vi "Configure PCM Settings.vi"(8 "error in":errorcluster, 11 "Measurement Configuration":T1={"Analog Source Resource Name"="", "IMD Standard"=0, "Custom Low Frequency"=14000.0, "Custom High frequency"=15000.0, "Custom Amplitude Ratio"=1.0, "Amplitude"=-1.0, "Protocol Source Resource Name"="7821\\PCMi 0", "Input range"=2.825, "Number of Words"=19200, "Clock Rate"=12288000, "Latch Delay"=0.0} {"Custom Amplitude Ratio" format="%.1f"; "Custom High frequency" format="%_2p"; "Custom Low Frequency" format="%#_2p"; "Clock Rate" format="%.4p"}) -> (0 "error out":errorcluster, 3 "PCM Input Task out":T2)   [LabVIEW 2021, in "audio_intermodulationDistortionMeasurement.lvlib"]
uses:
  audio_intermodulationDistortionMeasurement.lvlib
  <vilib>/PDM Acquisition Toolkit/host/Classes/Tasks/PCM Input/Controls/DVR PCM Input Task.ctl
  <vilib>/PDM Acquisition Toolkit/host/Classes/Tasks/PCM Input/PCM Input Task.lvclass
  <vilib>/PDM Acquisition Toolkit/host/Classes/Tasks/PDM Tasks/Controls/Acquisition Mode.ctl
  <vilib>/PDM Acquisition Toolkit/shared/controls/PCM Frame Sync Control.ctl
  <vilib>/PDM Acquisition Toolkit/shared/controls/Digital Edge.ctl
  <vilib>/PDM Acquisition Toolkit/shared/controls/PCM Data Format Configuration.ctl
  <vilib>/PDM Acquisition Toolkit/shared/controls/PCM Bit Endianness.ctl
  <vilib>/PDM Acquisition Toolkit/shared/controls/PCM Data Justification.ctl
  <vilib>/PDM Acquisition Toolkit/host/Classes/Session/Controls/Logic Levels.ctl
  <vilib>/PDM Acquisition Toolkit/host/API/Public/Create Tasks/Create PCM Input Task.vi
  <vilib>/PDM Acquisition Toolkit/host/API/Public/Configure/Timing/Configure Timing - PCM Input Slave.vi
  <vilib>/PDM Acquisition Toolkit/host/API/Public/Configure/PDM Channel/Configure Microphone Sensitivity FSPA - PCM Input Task.vi
  <vilib>/PDM Acquisition Toolkit/host/API/PDM Acquisition Toolkit.lvlib
  <vilib>/PDM Acquisition Toolkit/host/Classes/Tasks/PDM Tasks/PDM Task.lvclass
  <vilib>/PDM Acquisition Toolkit/shared/PDM Shared.lvlib
  <vilib>/PDM Acquisition Toolkit/host/Classes/Session/DecoderSession.lvclass
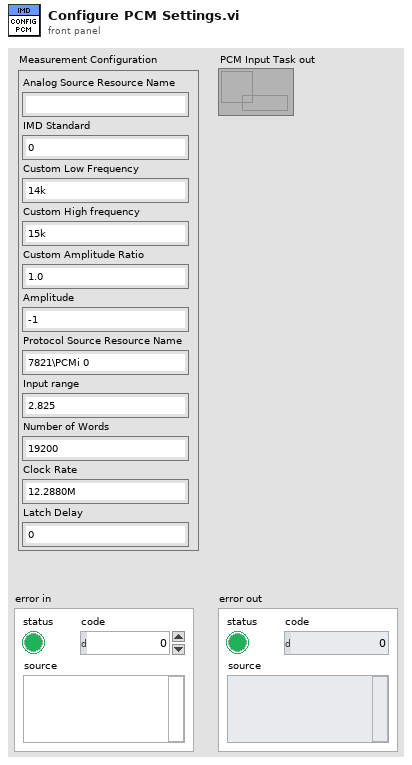
[diagram p1: front panel]
types:
  T1 = cluster{"Analog Source Resource Name":string, "IMD Standard":u16, "Custom Low Frequency":dbl, "Custom High frequency":dbl, "Custom Amplitude Ratio":dbl, "Amplitude":dbl, "Protocol Source Resource Name":string, "Input range":dbl, "Number of Words":i32, "Clock Rate":u32, "Latch Delay":dbl}
  T2 = typedef "PDM Acquisition Class Library.lvlib/PCM Input Task.lvclass/DVR PCM Input Task.ctl" = refnum<data-value>
  T3 = typedef "PDM Acquisition Class Library.lvlib/DecoderSession.lvclass/Logic Levels.ctl" = enum16{"3.3 V", "1.8 V", "1.2 V"}
  T4 = typedef "PDM Shared.lvlib/PCM Data Format Configuration.ctl" = cluster{"Frame Sync Edge for Channel 0":T5, "Channel Count Per Frame":u8, "Channel Length":u16, "Bit Depth":u8, "Channel 0 Offset":u16, "Endianness":T6, "Data Justification":T7}
  T5 = typedef "PDM Shared.lvlib/Digital Edge.ctl" = enum8{"Rising", "Falling"}
  T6 = typedef "PDM Shared.lvlib/PCM Bit Endianness.ctl" = enum16{"MSB First", "LSB First"}
  T7 = typedef "PDM Shared.lvlib/PCM Data Justification.ctl" = enum16{"Left Justified", "Right Justified"}
  T8 = typedef "PDM Shared.lvlib/PCM Frame Sync Control.ctl" = cluster{"Frame Length":u16, "Frame Sync Pulse Width":u16, "Bit Clock Edge  Sync":T5}
  T9 = typedef "PDM Acquisition Class Library.lvlib/PDM Task.lvclass/Acquisition Mode.ctl" = enum16{"Finite", "Continuous"}
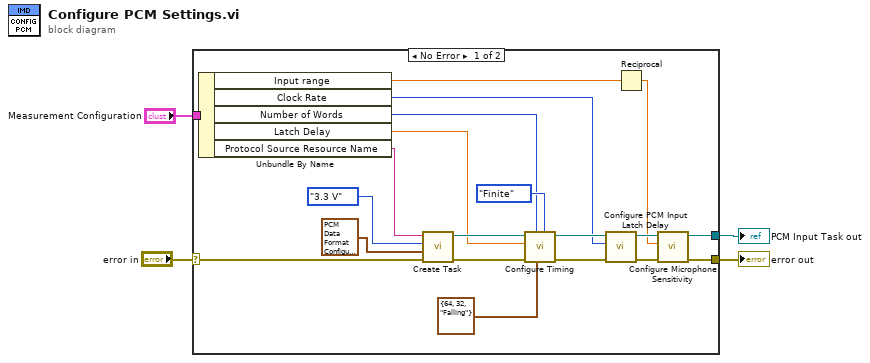
[diagram p0: block diagram]
diagram:
  n1 = case shown="No Error" "error in" {
    selector: "error in" -> [w23 w25]
    tunnel: [w7 w25] -> w3
    tunnel: "Measurement Configuration" -> [w24 _]
    tunnel: [w8 _] -> w2
    frame No Error {
      n2 = Unbundle By Name(w24) -> ("Input range"=w9:dbl, "Clock Rate"=w14:u32, "Number of Words"=w5:i32, "Latch Delay"=w6:dbl, "Protocol Source Resource Name"=w19:string)
      n3 = call-poly <vilib>:"Create Task.vi"("error in"=w23, "PCM data configuration"=T4 {"Frame Sync Edge for Channel 0"=enum."Falling", "Channel Count Per Frame"=2, "Channel Length"=32, "Bit Depth"=24, "Channel 0 Offset"=1, "Endianness"=enum."MSB First", "Data Justification"=enum."Left Justified"}, "logic level"=Logic_Levels."3.3 V", "channel list"=w19) -> ("error out"=w22:errorcluster, "PCM input task out"=w18:T2)  [unwired: 6 in]
      n4 = call-poly <vilib>:"Configure Timing.vi"("acquisition mode"=Acquisition_Mode."Finite", "Frame Sync Clock Control"=T8 {"Frame Length"=64, "Frame Sync Pulse Width"=32, "Bit Clock Edge  Sync"=enum."Falling"}, "number of words per channel"=w5, "error in"=w22, "Bit Clock rate"=w6, "PCM input task in"=w18) -> ("error out"=w21:errorcluster, "PCM input task out"=w17:T2)  [unwired: 4 in]
      n5 = call <vilib>:"Configure PCM Input Latch Delay.vi"("error in"=w21, "Latch Delay(ns)"=w14, "PCM input task in"=w17) -> ("error out"=w20:errorcluster, "PCM input task out"=w16:T2)  [unwired: 6 in, 1 out]
      n6 = Reciprocal(x=w9) -> (1/x=w10:dbl)
      n7 = call-poly <vilib>:"Configure Microphone Sensitivity.vi"("error in"=w20, "microphone sensitivity (FS/Pa)"=w10, "PCM input task in"=w16) -> ("error out"=w7:errorcluster, "PCM input task out"=w8:T2)  [unwired: 7 in]
    }
    frame Error {
    }
  }
  "error out" <- w3
  "PCM Input Task out" <- w2
